vi "define course periods.vi"(6 "periods per day":i32, 9 "expanded class data":bool[][](array[boolean]), 11 "Course ranking":i32[](array[numeric])) -> (2 "course periods":i32[](array[numeric]))   [LabVIEW 2009]
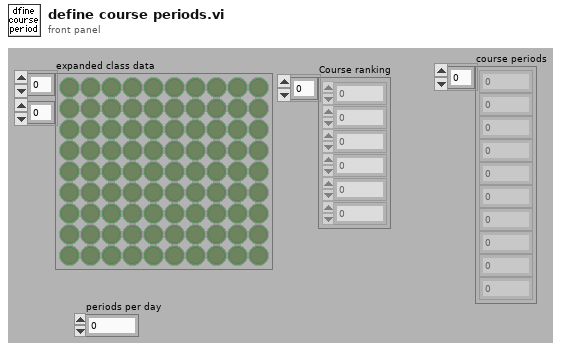
[diagram p1: front panel]
types:
  T1 = cluster{"class course ID":i32, "other index":i32, "rank":i32, "Acceptable solution":bool}[]
  T2 = cluster{"class course ID":i32, "other index":i32, "rank":i32, "Result":bool[]}
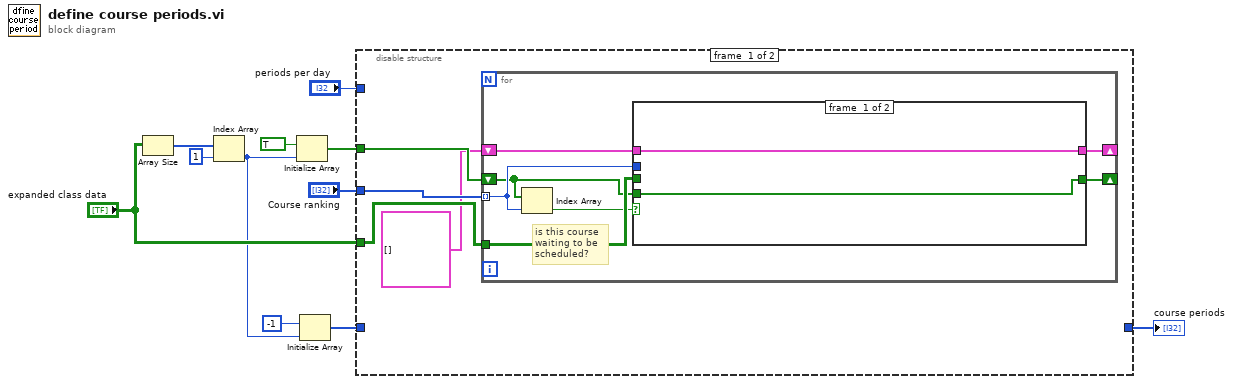
[diagram p0: block diagram]
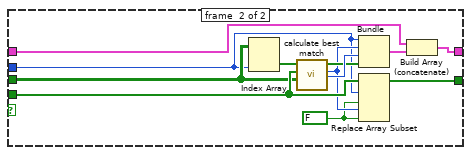
[diagram p2: hidden frame]
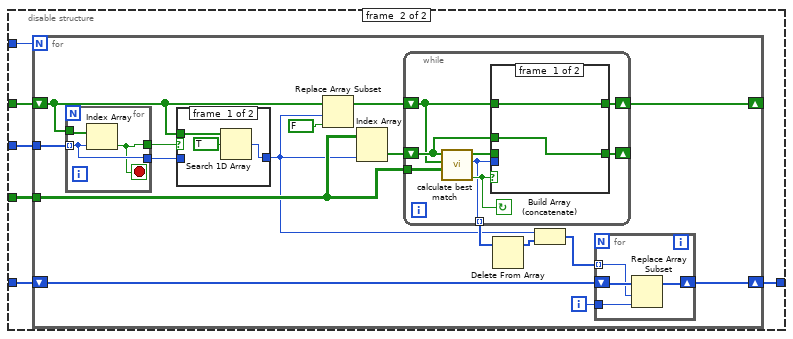
[diagram p3: hidden frame]
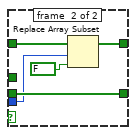
[diagram p5: hidden frame]
diagram:
  n1 = Array Size(array="expanded class data") -> (size(s)=w8:i32[])
  n2 = Index Array(array=w8, index=1) -> (element=w4:i32)
  n3 = Initialize Array(TRUE, w4) -> (w11:bool[])
  n4 = Initialize Array(-1 ("index"), w4) -> (w2:i32[])
  n5 = disable-structure shown="Enabled" {
    disable-tunnel: w11 -> [w15 w39]
    disable-tunnel: "expanded class data" -> [w14 w41]
    disable-tunnel: "Course ranking" -> [w13 w40]
    disable-tunnel: "periods per day" -> [_ w42]
    disable-tunnel: w2 -> [_ w38]
    disable-tunnel: [_ w37] -> w1
    frame #0 {
      n6 = for {
        tunnel: w14 -> [w22]
        tunnel: w13 -> [w19] mode=indexing
        shift-right: [w21] -> _
        shift-left: T1 [] -> [w20]
        shift-right: [w16] -> _
        shift-left: w15 -> [w17]
        # "is this course\nwaiting to be\nscheduled?"
        n7 = Index Array(array=w17, index=w19) -> (element=w18:bool)
        n8 = case shown="True" w18 {
          tunnel: w22 -> [_ w27]
          tunnel: [w24 w33] -> w21
          tunnel: w20 -> [w24 w32]
          tunnel: w19 -> [_ w25]
          tunnel: w17 -> [w23 w31]
          tunnel: [w23 w28] -> w16
          frame #0 {
          }
          frame #1 {
            w29 = FALSE
            n9 = Index Array(array=w27, index (col)=w25) -> (element=w26:bool[])  [unwired: 1 in]
            n10 = call "calculate best match.vi"("Array"=w27, "Allowed columns"=w31, "comparison"=w26) -> ("rank"=w36:i32, "other index"=w30:i32, "Result"=w35:bool[])  [unwired: 5 in, 1 out]
            n11 = Bundle("class course ID"=w25, "other index"=w30, "rank"=w36, "Result"=w35) -> (w34:T2)  [unwired: 1 in]
            n12 = Replace Array Subset(array=w31, new element #1=w29, index #1=w25, new element #2=w29, index #2=w30) -> (w28:bool[])
            n13 = Build Array (concatenate)(w32, w34) -> (w33:T1)
          }
        }
      }
    }
    frame #1 {
      n14 = for {
        N: w42 -> [_]
        tunnel: w41 -> [w52]
        tunnel: w40 -> [w58]
        shift-right: [w57] -> _
        shift-left: w39 -> [w54]
        shift-right: [w43] -> w37
        shift-left: w38 -> [w45]
        i -> [w44]
        n15 = for {
          tunnel: w54 -> [w69]
          tunnel: w58 -> [w68] mode=indexing
          tunnel: [w68] -> w55
          tunnel: [w67] -> w56
          stop <- w67 stop-if-true
          n16 = Index Array(array=w69, index=w68) -> (element=w67:bool)
        }
        n17 = case shown="False" w56 {
          tunnel: w54 -> [w65 _]
          tunnel: [w64 w66] -> w48
          tunnel: w55 -> [_ w66]
          frame #0 {
            n18 = Search 1D Array(1D array=w65, element=TRUE) -> (index of element=w64:i32)  [unwired: 1 in]
          }
          frame #1 {
          }
        }
        n19 = Replace Array Subset(array=w54, new element=FALSE ("new element/subarray"), index=w48) -> (w47:bool[])
        n20 = Index Array(array=w52, index (col)=w48) -> (element=w51:bool[])  [unwired: 1 in]
        n21 = while {
          shift-right: [w75] -> _
          shift-left: w51 -> [w73]
          tunnel: w52 -> [w77]
          shift-right: [w72] -> w57
          shift-left: w47 -> [w71]
          tunnel: [w70] -> w50 mode=indexing
          stop <- w76 continue-if-true
          n22 = call "calculate best match.vi"("Array"=w77, "Allowed columns"=w71, "comparison"=w73) -> ("Acceptable solution"=w76:bool, "other index"=w70:i32, "Result"=w74:bool[])  [unwired: 5 in, 1 out]
          n23 = case shown="True" w76 {
            tunnel: [w79 w84] -> w75
            tunnel: w74 -> [_ w84]
            tunnel: w73 -> [w79 _]
            tunnel: w70 -> [_ w81]
            tunnel: [w78 w82] -> w72
            tunnel: w71 -> [w78 w83]
            frame #0 {
            }
            frame #1 {
              n24 = Replace Array Subset(array=w83, new element=FALSE ("new element/subarray"), index=w81) -> (w82:bool[])
            }
          }
        }
        n25 = Delete From Array(array=w50) -> (array with subset deleted=w49:i32[])  [unwired: 2 in, 1 out]
        n26 = Build Array (concatenate)(w48, w49) -> (w46:i32[])
        n27 = for {
          tunnel: w46 -> [w61] mode=indexing
          shift-right: [w60] -> w43
          shift-left: w45 -> [w62]
          tunnel: w44 -> [w59]
          n28 = Replace Array Subset(array=w62, new element=w59, index=w61) -> (w60:i32[])
        }
      }
    }
  }
  "course periods" <- w1
